vi "Status.vi"(8 "error in (no error)":errorcluster, 11 "Response Core in":refnum<class "Response Core.lvclass">) -> (0 "error out":errorcluster, 1 "Time to Timeout (ms)":i32, 2 "Dropped?":bool, 3 "Response Core out":refnum<class "Response Core.lvclass">)   [LabVIEW 2020, in "Publisher.lvlib" / "Response Core.lvclass"]
doc: "Check if the Response Core has been dropped."
uses:
  Response Core.lvclass
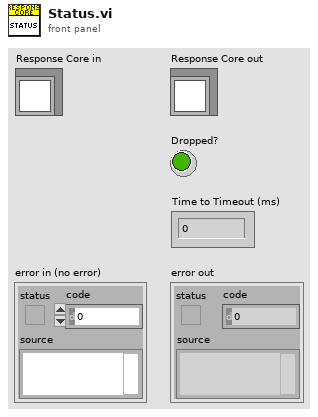
[diagram p1: front panel]
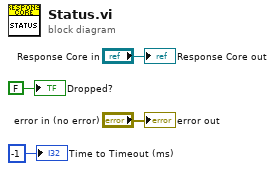
[diagram p0: block diagram]
diagram:
  "error out" <- "error in (no error)"
  "Response Core out" <- "Response Core in"
  "Dropped?" <- FALSE ("Dropped?")
  "Time to Timeout (ms)" <- -1 ("Time to Timeout (ms)")
